vi "ReadStartupBehavior.vi"(8 "error in (no error)":errorcluster, 11 "SMO in":refnum<class "SMO.lvclass">) -> (0 "error out":errorcluster, 2 "Behavior":T1, 3 "SMO out":refnum<class "SMO.lvclass">)   [LabVIEW 2019, in "SMO.lvclass"]
doc: "JKI State Machine Objects (SMO) 1.3.0.56\nJKI - JKI\nCopyright (c) 2017, JKI"
uses:
  SMO.lvclass
  Support/Attribute.StartupBehavior/ProcessStartupBehavior.ctl
  Support/Attribute/Attribute.lvclass
  Support/Attribute.StartupBehavior/Attribute.StartupBehavior.lvclass
  C:/Users/Patrick/Documents/GitHub/Test (LV2019)/lv-venv/lv.lib/vi.lib/JKI/JKI SMO/Support/Attribute/Attribute.lvclass
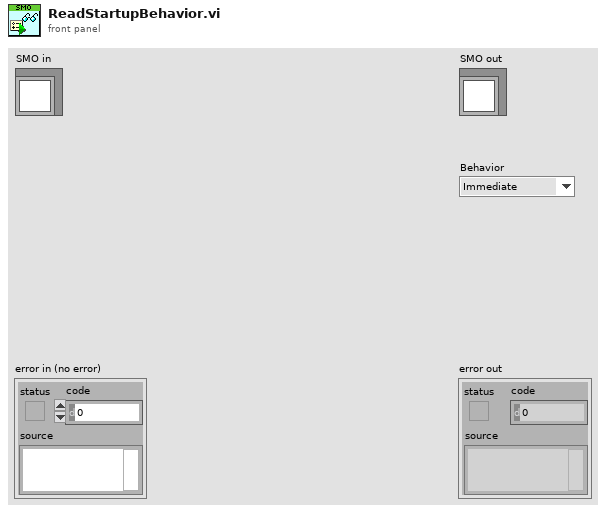
[diagram p1: front panel]
types:
  T1 = typedef "Attribute.StartupBehavior.lvclass/ProcessStartupBehavior.ctl" = enum16{"Immediate", "First Call", "Never"}
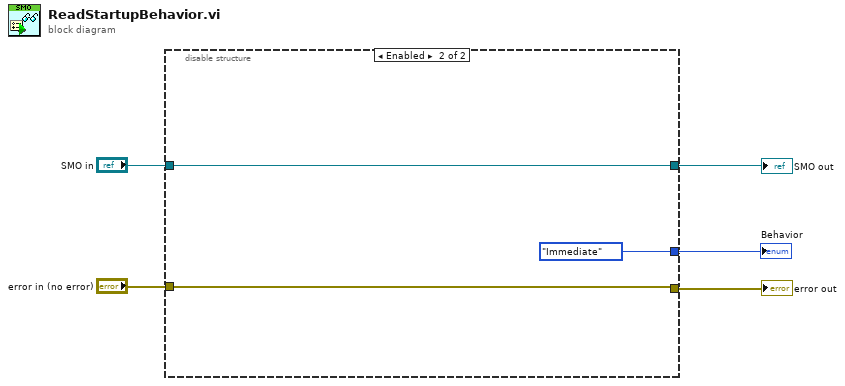
[diagram p0: block diagram]
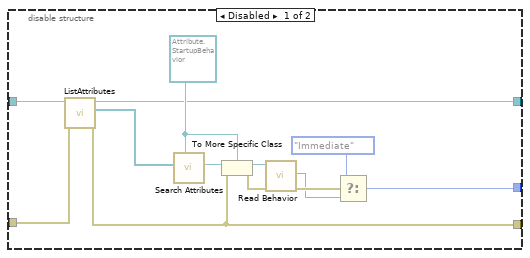
[diagram p2: hidden frame]
diagram:
  n1 = disable-structure shown="Enabled" {
    disable-tunnel: "SMO in" -> [w16 w20]
    disable-tunnel: "error in (no error)" -> [w15 w19]
    disable-tunnel: [w13 w20] -> w3
    disable-tunnel: [w12 w19] -> w2
    disable-tunnel: [w6 ProcessStartupBehavior."Immediate" ("t")] -> w1
    frame Disabled {
      w14 = refnum<class "Attribute.StartupBehavior.lvclass"> refnum ("Attribute.StartupBehavior.lvclass")
      n2 = call "ListAttributes.vi"("error in (no error)"=w15, "SMO in"=w16) -> ("error out"=w12:errorcluster, "[Attributes]"=w17:refnum<class "Attribute.lvclass">[], "SMO out"=w13:refnum<class "SMO.lvclass">)  [unwired: 7 in]
      n3 = call "Search Attributes.vi"("Attribute type"=w14, "[Attributes]"=w17) -> ("Attribute out"=w18:refnum<class "Attribute.lvclass">)  [unwired: 8 in, 1 out]
      n4 = To More Specific Class(target class=w14, reference=w18, error in=w12) -> (specific class reference=w11:refnum<class "Attribute.StartupBehavior.lvclass">, error out=w10:errorcluster)
      n5 = call "Read Behavior.vi"("error in (no error)"=w10, "Attribute.StartupBehavior in"=w11) -> ("error out"=w9:errorcluster, "Behavior"=w8:T1)  [unwired: 7 in, 1 out]
      n6 = Select(t=ProcessStartupBehavior."Immediate", s=w9, f=w8) -> (s? t:f=w6:T1)
    }
    frame Enabled {
    }
  }
  "error out" <- w2
  "SMO out" <- w3
  "Behavior" <- w1
